vi "Register for gRPC Server Events.vi"(8 "error in (no error)":errorcluster, 11 "CIFLauncher in":refnum<class "CIFLauncher.lvclass">) -> (0 "error out":errorcluster, 2 "Event Registration Refnum":refnum<event-registration>, 3 "CIFLauncher out":refnum<class "CIFLauncher.lvclass">)   [LabVIEW 2021, in "CIFLauncher.lvclass"]
uses:
  CIFLauncher.lvclass
  CIF_Launcher_server/RPC Service/Launcher/Launcher.lvclass
  C:/Program Files/National Instruments/LabVIEW 2021/vi.lib/gRPC/LabVIEW gRPC Servicer/ServiceBase/ServiceBase.lvclass
  CIF_Launcher_server/RPC Service/Launcher/Launcher.lvclass/Launcher.ctl
  CIFLauncher.lvclass/CIFLauncher.ctl
  D:/dev/CIF-LVCore/src/CIFPluginManager/CIFLauncher/gRPC/CIF_Launcher_server/RPC Service/Launcher/Launcher.lvclass
  <vilib>/gRPC/LabVIEW gRPC Library/Shared/grpcId.ctl
  <vilib>/gRPC/LabVIEW gRPC Library/grpc-lvsupport-release.lvlib
  <vilib>/gRPC/LabVIEW gRPC Library/Server API/typeDefs/gRPCId Cluster.ctl
  CIF_Launcher_server/RPC Service/Launcher/typeDefs/Server gRPC UEs.ctl
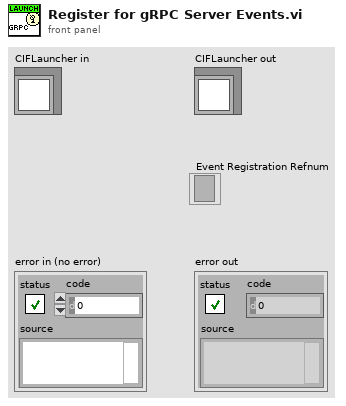
[diagram p1: front panel]
types:
  T1 = typedef "CIF_Launcher_server.lvlib/Launcher.lvclass/Server gRPC UEs.ctl" = cluster{"Launcher LaunchPlugin gRPC UE":refnum<user-event>, "Launcher AbortPlugin gRPC UE":refnum<user-event>, "Launcher Destroy gRPC UE":refnum<user-event>, "Launcher Ping gRPC UE":refnum<user-event>, "Launcher Discover gRPC UE":refnum<user-event>}
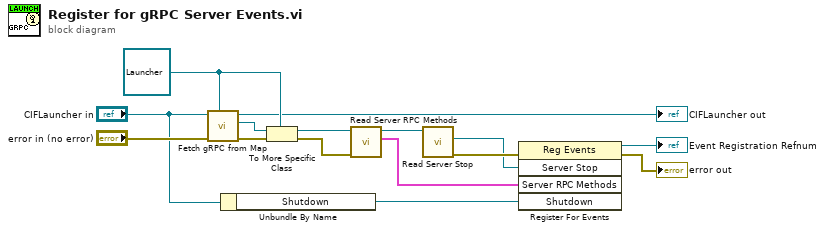
[diagram p0: block diagram]
diagram:
  w13 = refnum<class "Launcher.lvclass"> refnum ("CIF_Launcher_server.lvlib:Launcher.lvclass")
  n1 = call "Fetch gRPC from Map.vi"("gRPC Server Class type"=w13, "error in (no error)"="error in (no error)", "CIFLauncher in"="CIFLauncher in") -> ("error out"=w12:errorcluster, "gRPC Server Class out"=w14:refnum<class "ServiceBase.lvclass">, "CIFLauncher out"=→"CIFLauncher out":refnum<class "CIFLauncher.lvclass">)  [unwired: 6 in]
  n2 = Unbundle By Name("CIFLauncher in") -> ("Shutdown"=w2:refnum<user-event>)
  n3 = To More Specific Class(target class=w13, reference=w14, error in=w12) -> (specific class reference=w6:refnum<class "Launcher.lvclass">, error out=w10:errorcluster)
  n4 = call "Read Server RPC Methods.vi"("error in (no error)"=w10, "SignalGeneratorService in"=w6) -> ("Server RPC Methods"=w7:T1, "SignalGeneratorService out"=w15:refnum<class "Launcher.lvclass">)  [unwired: 7 in, 1 out]
  n5 = call-dynamic "Read Server Stop.vi"("iService in"=w15) -> ("error out"=w9:errorcluster, "Server Stop"=w8:refnum<user-event>)  [unwired: 8 in, 1 out]
  n6 = register-events(error in=w9, w8, w7, w2) -> (reference out=→"Event Registration Refnum":refnum<event-registration>, error out=→"error out":errorcluster)  [unwired: 1 in]
